vi "Insert Line Into File.vi"(7 "Check Only? (f)":bool, 8 "Error In":errorcluster, 9 "Line":string="i2c-bcm2708", 10 "File Path":string="cat /etc/modules", 11 "Install LV Data":T1={"SSH Session"=refnum, "Status Log"="", "Detailed Log"="", "Credentials"={"Hostname or IP"="192.168.7.2", "Username"="root", "Password"=""}, "Target Info"={"OS Version"="", "CPU"="", "Systemd Version"="", "Internet Access"=FALSE, "Device Type"="", "LV Installed Ver"="", "LV Available Ver"="", "LV Upgrade Available"=FALSE, "Hostname"="", "NIC Info"=[]}, "Reboot Required?"=FALSE}) -> (0 "Error Out":errorcluster, 1 "Log":string, 2 "Line Alredy Present?":bool, 3 "Install LV Data":T1={"SSH Session"=refnum, "Status Log"="", "Detailed Log"="", "Credentials"={"Hostname or IP"="192.168.7.2", "Username"="root", "Password"=""}, "Target Info"={"OS Version"="", "CPU"="", "Systemd Version"="", "Internet Access"=FALSE, "Device Type"="", "LV Installed Ver"="", "LV Available Ver"="", "LV Upgrade Available"=FALSE, "Hostname"="", "NIC Info"=[]}, "Reboot Required?"=FALSE})   [LabVIEW 2020, in "LMH-LINX.lvlib"]
uses:
  LMH-LINX.lvlib
  Install LV Data.ctl
  Target Info.ctl
  NIC Info.ctl
  NIC Mode.ctl
  <vilib>/regexp/Match Regular Expression.xnode
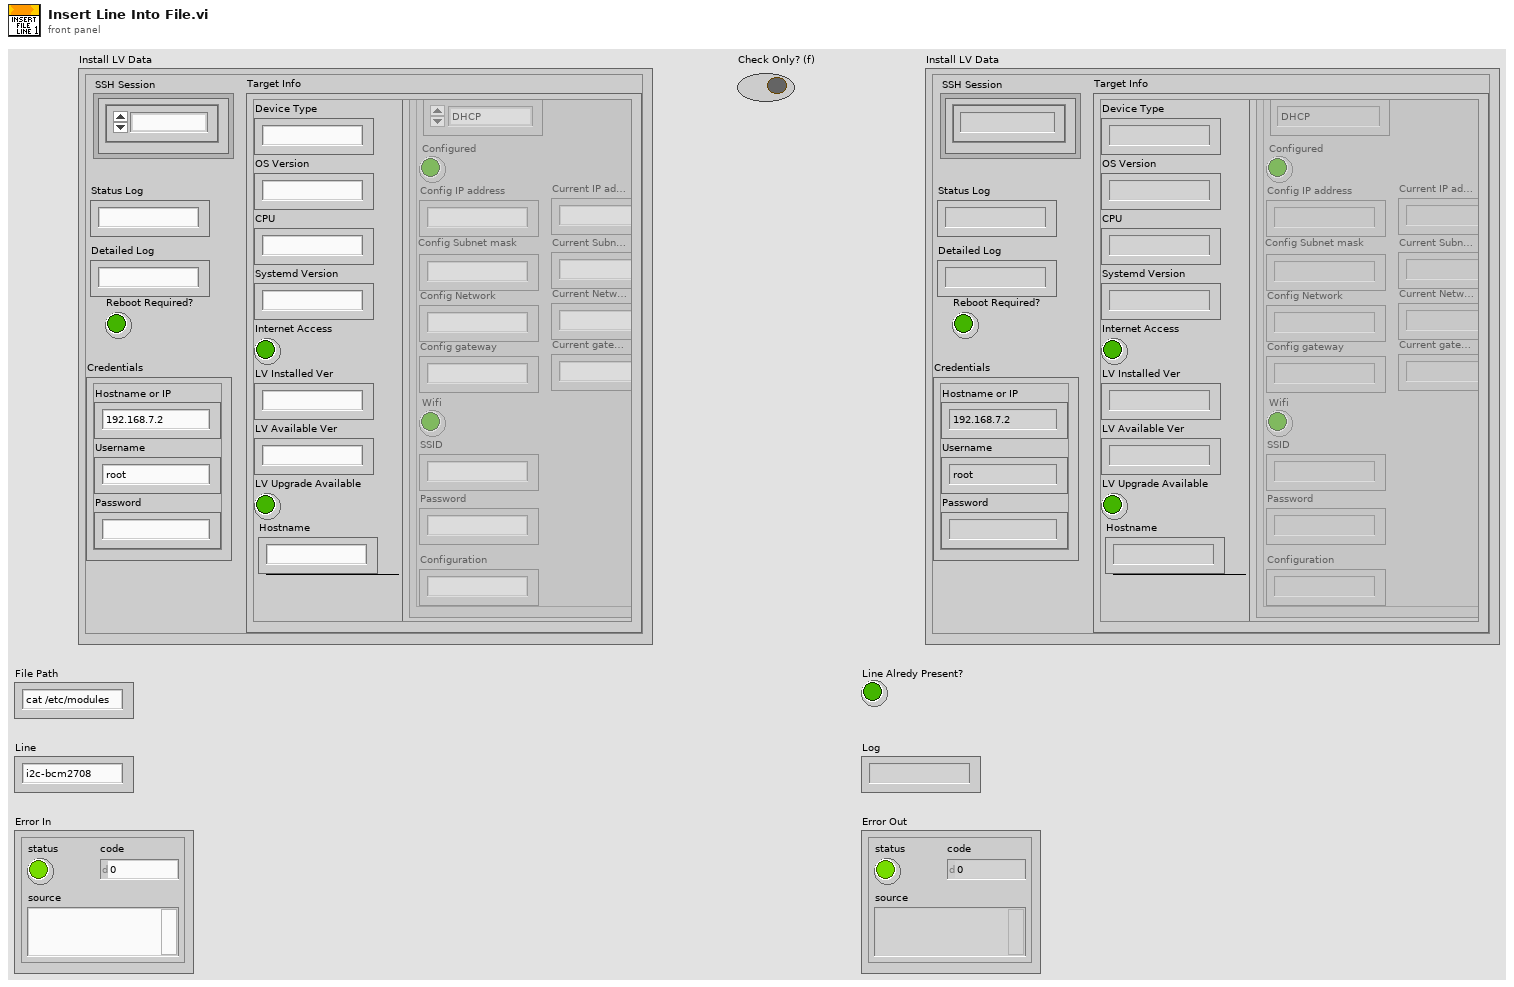
[diagram p1: front panel]
types:
  T1 = typedef "LMH-LINX.lvlib/Install LV Data.ctl" = cluster{"SSH Session":refnum<k1>, "Status Log":string, "Detailed Log":string, "Credentials":cluster{"Hostname or IP":string, "Username":string, "Password":string}, "Target Info":T2, "Reboot Required?":bool}
  T2 = typedef "LMH-LINX.lvlib/Target Info.ctl" = cluster{"OS Version":string, "CPU":string, "Systemd Version":string, "Internet Access":bool, "Device Type":string, "LV Installed Ver":string, "LV Available Ver":string, "LV Upgrade Available":bool, "Hostname":string, "NIC Info":T3[]}
  T3 = typedef "LMH-LINX.lvlib/NIC Info.ctl" = cluster{"Name":string, "NIC Mode":T4, "Configured":bool, "Config IP address":string, "Config Subnet mask":string, "Config Network":string, "Config gateway":string, "Wifi":bool, "SSID":string, "Password":string, "Configuration":string, "Current IP address":string, "Current Subnet mask":string, "Current gateway":string, "Current Network":string}
  T4 = typedef "LMH-LINX.lvlib/NIC Mode.ctl" = enum16{"DHCP", "Static", "Loopback"}
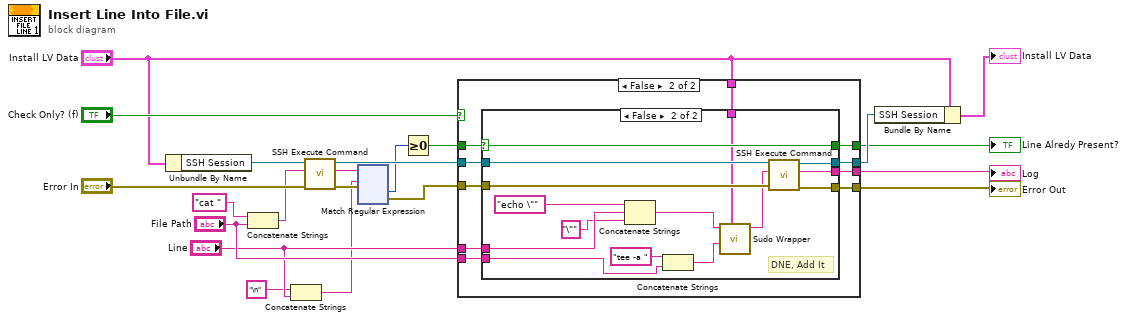
[diagram p0: block diagram]
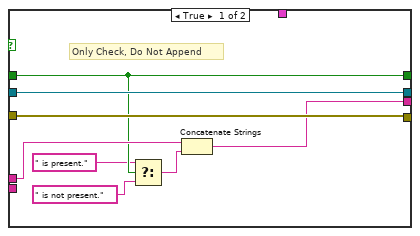
[diagram p2: hidden frame]
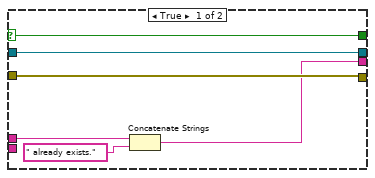
[diagram p3: hidden frame]
diagram:
  n1 = Unbundle By Name("Install LV Data") -> ("SSH Session"=w20:refnum<k1>)
  n2 = Concatenate Strings("cat " ("string"), "File Path") -> (w11:string)
  n3 = Concatenate Strings("\n", "Line") -> (w3:string)
  n4 = call "SSH Execute Command.vi"("Error In"="Error In", "Command"=w11, "SSH Session"=w20) -> ("Error Out"=w17:errorcluster, "Std Out"=w13:string, "SSH Session"=w18:refnum<k1>)  [unwired: 6 in]
  n5 = xnode "Match Regular Expression"("input string"=w13, "regular expression"=w3, "error in"=w17) -> ("offset past match"=w15:i32, "error out"=w16:errorcluster)  [unwired: 3 in, 3 out]
  n6 = Greater Or Equal To 0?(x=w15) -> (x >= 0?=w14:bool)
  n7 = case shown="False" "Check Only? (f)" {
    tunnel: w18 -> [w29 w39]
    tunnel: w16 -> [w28 w38]
    tunnel: w14 -> [w25 w37]
    tunnel: "Line" -> [w26 w36]
    tunnel: [w28 w35] -> w10
    tunnel: [w27 w34] -> w9
    tunnel: [w29 w33] -> w8
    tunnel: "File Path" -> [_ w32]
    tunnel: [w25 w31] -> w5
    tunnel: "Install LV Data" -> [_ w30]
    frame True {
      # "Only Check, Do Not Append"
      n8 = Select(t=" is present.", s=w25, f=" is not present.") -> (s? t:f=w22:string)
      n9 = Concatenate Strings(w26, w22) -> (w27:string)
    }
    frame False {
      n10 = case shown="False" w37 {
        selector: w37 -> [w40 w52]
        tunnel: [w41 w60] -> w34
        tunnel: [w45 w59] -> w35
        tunnel: [w44 w58] -> w33
        tunnel: w39 -> [w44 w57]
        tunnel: w38 -> [w45 w56]
        tunnel: w36 -> [w43 w54]
        tunnel: w32 -> [_ w47]
        tunnel: [w40 w52] -> w31
        tunnel: w30 -> [_ w46]
        frame True {
          n11 = Concatenate Strings(w43, " already exists." ("Std Out")) -> (w41:string)
        }
        frame False {
          # "DNE, Add It"
          n12 = Concatenate Strings("echo \"", w54, "\"" ("string")) -> (w48:string)
          n13 = Concatenate Strings("tee -a " ("string"), w47) -> (w49:string)
          n14 = call "Sudo Wrapper.vi"("Install LV Data"=w46, "comand string"=w49, "echo string"=w48) -> ("combined command string"=w51:string)  [unwired: 8 in]
          n15 = call "SSH Execute Command.vi"("Error In"=w56, "Command"=w51, "SSH Session"=w57) -> ("Error Out"=w59:errorcluster, "Std Out"=w60:string, "SSH Session"=w58:refnum<k1>)  [unwired: 6 in]
        }
      }
    }
  }
  "Log" <- w9
  "Error Out" <- w10
  "Line Alredy Present?" <- w5
  n16 = Bundle By Name(cluster="Install LV Data", "SSH Session"=w8) -> (→"Install LV Data":T1)
